vi "getNoShowMachine.vi"() -> (0 "rows":i32, 2 "Machine":string)   [LabVIEW 2012]
uses:
  <vilib>/addons/database/Connection.llb/DB Tools Open Connec (Path).vi
  <vilib>/addons/database/Connection.llb/Conn Execute.vi
  <vilib>/addons/database/Recordset.llb/Rec Fetch Recordset Data (R).vi
  <vilib>/addons/database/Recordset.llb/Rec Destroy - Connection.vi
  <vilib>/addons/database/_DB Variant To Data/Database Variant To Data.xnode
  <vilib>/addons/database/NI_Database_API.lvlib
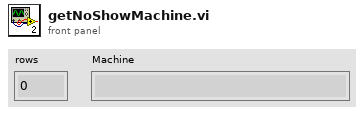
[diagram p1: front panel]
types:
  T1 = typedef "NI_Database_API.lvlib/Conn ObjectReference.ctl" = refnum<k1>
  T2 = typedef "NI_Database_API.lvlib/Rec ObjectReference.ctl" = refnum<k1>
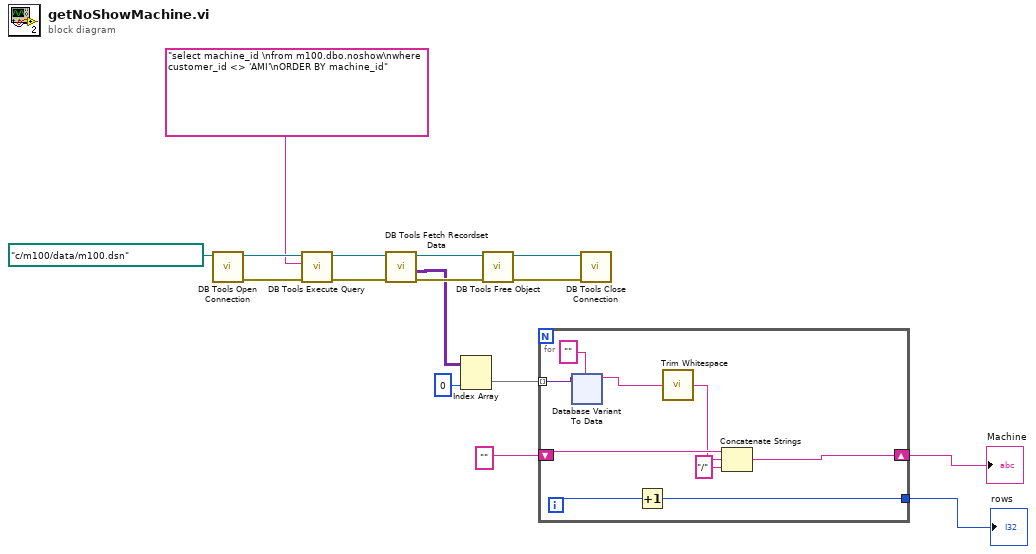
[diagram p0: block diagram]
diagram:
  n1 = call-poly <vilib>:"DB Tools Open Connection.vi"("connection information"=path "c:/m100/data/m100.dsn") -> ("error out"=w9:errorcluster, "connection reference"=w13:T1)  [unwired: 7 in]
  n2 = call-poly <vilib>:"DB Tools Execute Query.vi"("error in (no error)"=w9, "SQL query"="select machine_id \nfrom m100.dbo.noshow\nwhere customer_id <> 'AMI'\nORDER BY machine_id", "connection reference"=w13) -> ("error out"=w10:errorcluster, "recordset reference"=w14:T2)  [unwired: 5 in]
  n3 = call-poly <vilib>:"DB Tools Fetch Recordset Data.vi"("error in (no error)"=w10, "recordset reference"=w14) -> ("error out"=w11:errorcluster, "recordset data"=w6:variant[][], "recordset reference out"=w15:T2)  [unwired: 3 in]
  n4 = Index Array(array=w6, index (col)=0 ("disabled index (col)")) -> (element=w4:variant[])  [unwired: 1 in]
  n5 = call-poly <vilib>:"DB Tools Free Object.vi"("error in (no error)"=w11, "recordset reference"=w15) -> ("error out"=w12:errorcluster, "connection reference"=w16:T1)  [unwired: 8 in]
  n6 = for {
    tunnel: w4 -> [w25] mode=indexing
    shift-right: [w22] -> w2
    shift-left: "" ("string") -> [w24]
    tunnel: [w17] -> w1
    i -> [w18]
    n7 = xnode "Database Variant To Data"("database variant"=w25, "type"="") -> ("data"=w20:string)  [unwired: 1 in, 1 out]
    n8 = Increment(x=w18) -> (x+1=w17:i32)
    n9 = call <vilib>:"Trim Whitespace.vi"("string"=w20) -> ("trimmed string"=w21:string)  [unwired: 1 in]
    n10 = Concatenate Strings(w24, w21, "/" ("string")) -> (w22:string)
  }
  "Machine" <- w2
  "rows" <- w1
  n11 = call <vilib>:"DB Tools Close Connection.vi"("error in (no error)"=w12, "connection reference"=w16) -> ()  [unwired: 5 in, 1 out]
